vi "RSZVB Get Calibration Connection.vi"(8 "error in (no error)":errorcluster {"code" format="%.0x"}, 10 "Channel (1)":i32=1, 11 "VISA session":refnum<visa-resource-name>) -> (0 "error out":errorcluster {"code" format="%.0x"}, 1 "Analyzer Port 3":i32, 2 "Analyzer Port 2":i32, 3 "dup VISA session":refnum<visa-resource-name>, 4 "Analyzer Port 4":i32, 5 "Analyzer Port 1":i32)   [LabVIEW 2011]
doc: "This VI returns the assignment between the network analyzer ports and the ports of the connected automatic calibration unit. \n\nRemote-control command(s):\n[SENSe<Ch>:]CORRection:COLLect:AUTO:PORTs:CONNection?"
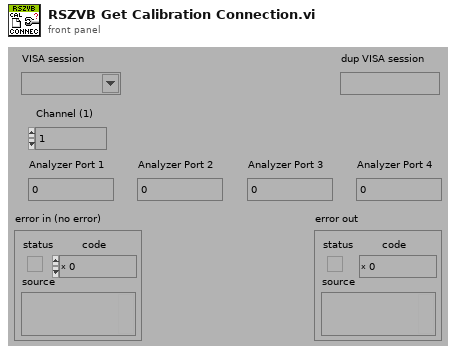
[diagram p1: front panel]
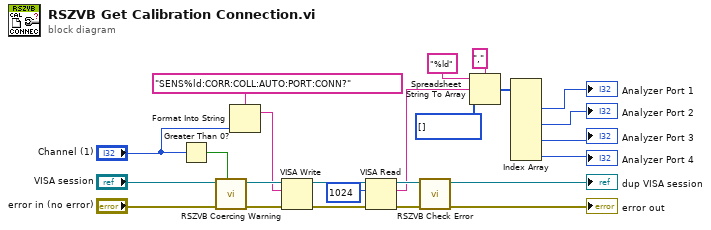
[diagram p0: block diagram]
diagram:
  n1 = Greater Than 0?(x="Channel (1)") -> (x > 0?=w15:bool)
  n2 = call "RSZVB Coercing Warning.vi"("In Range?"=w15, "error in (no error)"="error in (no error)", "VISA session"="VISA session") -> ("error out"=w22:errorcluster, "dup VISA session"=w23:refnum<visa-resource-name>)  [unwired: 7 in]
  n3 = Format Into String(format string="SENS%ld:CORR:COLL:AUTO:PORT:CONN?", "Channel (1)") -> (resulting string=w21:string)  [unwired: 2 in, 1 out]
  n4 = VISA Write(VISA resource name=w23, write buffer=w21, error in (no error)=w22) -> (VISA resource name out=w17:refnum<visa-resource-name>, error out=w16:errorcluster)  [unwired: 1 out]
  n5 = VISA Read(VISA resource name=w17, byte count=u32 1024 ("byte count (0)"), error in (no error)=w16) -> (VISA resource name out=w19:refnum<visa-resource-name>, read buffer=w9:string, error out=w18:errorcluster)  [unwired: 1 out]
  n6 = call "RSZVB Check Error.vi"("error in (no error)"=w18, "VISA session"=w19) -> ("error out"=→"error out":errorcluster, "dup VISA session"=→"dup VISA session":refnum<visa-resource-name>)  [unwired: 8 in]
  n7 = Spreadsheet String To Array(delimiter (Tab)=",", format string="%ld", spreadsheet string=w9, array type (2D Dbl)=i32[] []) -> (array=w1:i32[])
  n8 = Index Array(array=w1) -> (element #2=→"Analyzer Port 1":i32, element #4=→"Analyzer Port 2":i32, element #6=→"Analyzer Port 3":i32, element #8=→"Analyzer Port 4":i32)  [unwired: 8 in, 4 out]
